vi "get_video_codec_default_bitrate.vi"(8 "profile":u8, 9 "framerate":u8, 10 "height":u16, 11 "width":u16) -> (3 "bitrate":u32)   [LabVIEW 2023]
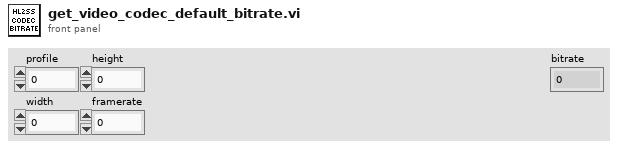
[diagram p1: front panel]
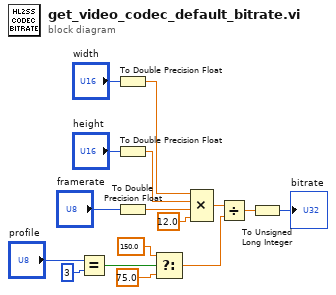
[diagram p0: block diagram]
diagram:
  n1 = Equal?(x="profile", y=u8 3) -> (x = y?=w10:bool)
  n2 = To Double Precision Float(number="width") -> (double precision float=w16:dbl)
  n3 = To Double Precision Float(number="height") -> (double precision float=w15:dbl)
  n4 = To Double Precision Float(number="framerate") -> (double precision float=w14:dbl)
  n5 = Select(t=150.0 ("y"), s=w10, f=75.0 ("t")) -> (s? t:f=w11:dbl)
  n6 = Compound Arithmetic op=MULTIPLY(w16, w15, w14, 12.0 ("value")) -> (w12:dbl)
  n7 = Divide(x=w12, y=w11) -> (x/y=w2:dbl)
  n8 = To Unsigned Long Integer(number=w2) -> (unsigned 32bit integer=→"bitrate":u32)
